vi "Homing.vi"() -> ()   [LabVIEW 2013]
panel:
  in  "MG17Motor 5":refnum<k7>(container)
  in  "MG17Motor 4":refnum<k7>(container)
  in  "MG17Motor 3":refnum<k7>(container)
  in  "Serial 3":i32=90848557
  in  "Serial 2":i32=90848557
  in  "Serial":i32=90848557
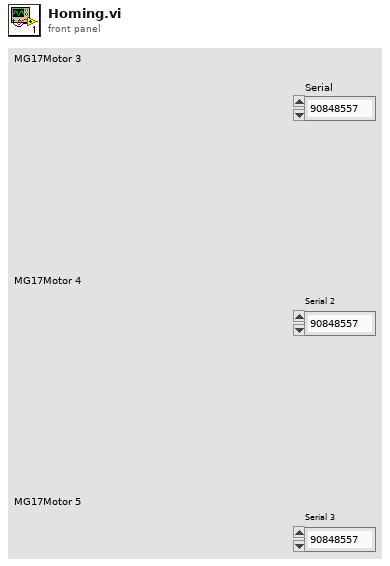
[diagram p1: front panel]
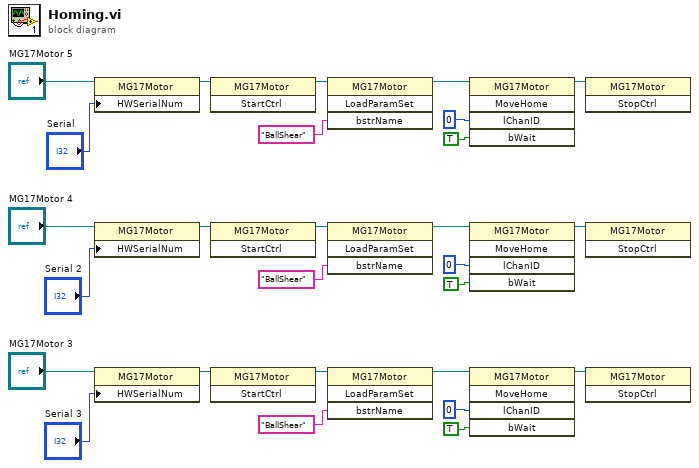
[diagram p0: block diagram]
diagram:
  n1 = property class="MG17Motor"(reference="MG17Motor 5", "HWSerialNum"="Serial") -> (reference out=w26:refnum<k7>)  [unwired: 1 in, 1 out]
  n2 = property class="MG17Motor"(reference="MG17Motor 4", "HWSerialNum"="Serial 2") -> (reference out=w18:refnum<k7>)  [unwired: 1 in, 1 out]
  n3 = property class="MG17Motor"(reference="MG17Motor 3", "HWSerialNum"="Serial 3") -> (reference out=w10:refnum<k7>)  [unwired: 1 in, 1 out]
  n4 = invoke class="MG17Motor" method="StartCtrl"(reference=w26) -> (reference out=w23:refnum<k7>)  [unwired: 2 in, 2 out]
  n5 = invoke class="MG17Motor" method="StartCtrl"(reference=w18) -> (reference out=w15:refnum<k7>)  [unwired: 2 in, 2 out]
  n6 = invoke class="MG17Motor" method="StartCtrl"(reference=w10) -> (reference out=w7:refnum<k7>)  [unwired: 2 in, 2 out]
  n7 = invoke class="MG17Motor" method="LoadParamSet"(reference=w23, "bstrName"="BallShear") -> (reference out=w21:refnum<k7>)  [unwired: 2 in, 3 out]
  n8 = invoke class="MG17Motor" method="LoadParamSet"(reference=w15, "bstrName"="BallShear") -> (reference out=w13:refnum<k7>)  [unwired: 2 in, 3 out]
  n9 = invoke class="MG17Motor" method="LoadParamSet"(reference=w7, "bstrName"="BallShear") -> (reference out=w5:refnum<k7>)  [unwired: 2 in, 3 out]
  n10 = invoke class="MG17Motor" method="MoveHome"(reference=w21, "lChanID"=0, "bWait"=TRUE) -> (reference out=w24:refnum<k7>)  [unwired: 2 in, 4 out]
  n11 = invoke class="MG17Motor" method="MoveHome"(reference=w13, "lChanID"=0, "bWait"=TRUE) -> (reference out=w16:refnum<k7>)  [unwired: 2 in, 4 out]
  n12 = invoke class="MG17Motor" method="MoveHome"(reference=w5, "lChanID"=0, "bWait"=TRUE) -> (reference out=w8:refnum<k7>)  [unwired: 2 in, 4 out]
  n13 = invoke class="MG17Motor" method="StopCtrl"(reference=w24) -> ()  [unwired: 2 in, 3 out]
  n14 = invoke class="MG17Motor" method="StopCtrl"(reference=w16) -> ()  [unwired: 2 in, 3 out]
  n15 = invoke class="MG17Motor" method="StopCtrl"(reference=w8) -> ()  [unwired: 2 in, 3 out]
